vi "Crossover v2.vi"(10 "Path In 2":T1={"Distance"=0.0, "Tour"=[1, 8, 6, 10, 4, 13, 16, 2, 3, 12, 15, 5, 9, 11, 14, 7, 1]}, 11 "Path In 1":T1={"Distance"=0.0, "Tour"=[1, 14, 13, 12, 7, 6, 15, 5, 11, 9, 10, 16, 3, 2, 4, 8, 1]}) -> (2 "Path Out 2":T1, 3 "Path Out 1":T1)   [LabVIEW 2015, in "TSP Library.lvlib"]
uses:
  TSP Library.lvlib
  TypeDef/Path.ctl
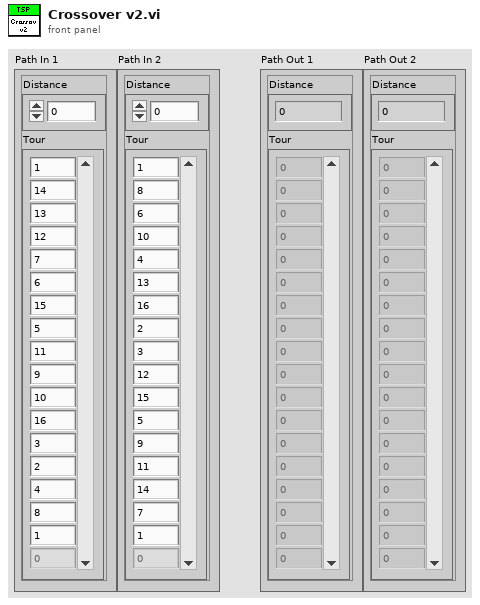
[diagram p1: front panel]
types:
  T1 = typedef "TSP Library.lvlib/Path.ctl" = cluster{"Distance":dbl, "Tour":u16[]}
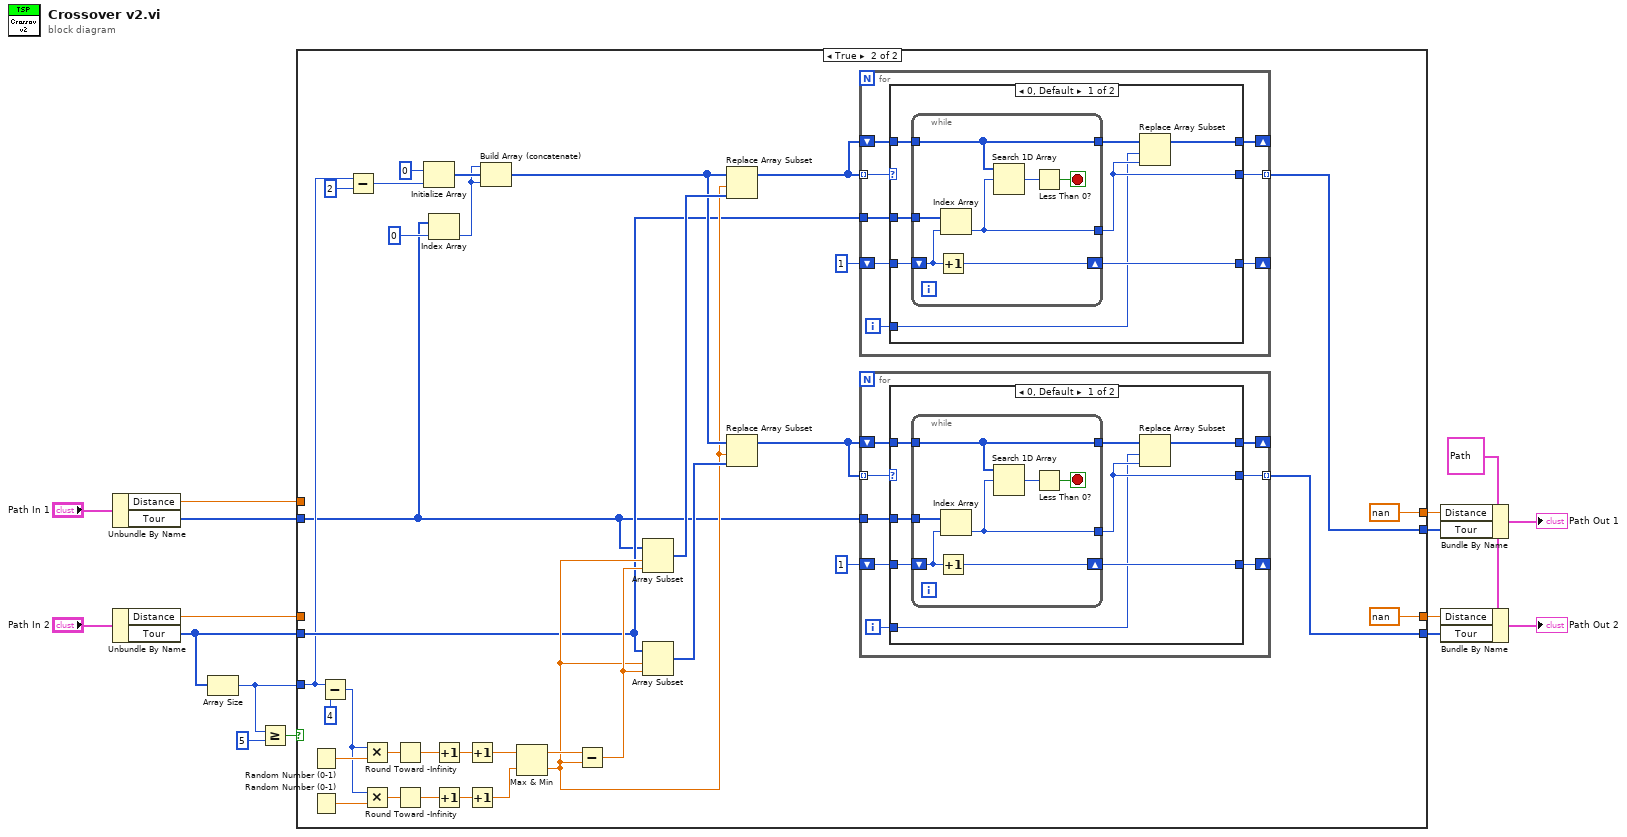
[diagram p0: block diagram]
diagram:
  w9 = T1 {"Distance"=0.0, "Tour"=[68, 82, 14, 66, 38, 76, 91, 89, 87, 84, 25, 25, 88]} ("Path In 1")
  n1 = Unbundle By Name("Path In 1") -> ("Distance"=w11:dbl, "Tour"=w12:u16[])
  n2 = Unbundle By Name("Path In 2") -> ("Distance"=w13:dbl, "Tour"=w14:u16[])
  n3 = Array Size(array=w14) -> (size(s)=w2:i32)
  n4 = Greater Or Equal?(x=w2, y=5) -> (x >= y?=w3:bool)
  n5 = case shown="True" w3 {
    tunnel: w2 -> [_ w27]
    tunnel: w14 -> [w17 w30]
    tunnel: w13 -> [w18 _]
    tunnel: w12 -> [w19 w22]
    tunnel: w11 -> [w20 _]
    tunnel: [w19 w25] -> w7
    tunnel: [w17 w21] -> w6
    tunnel: [w18 nan ("Distance")] -> w5
    tunnel: [w20 nan ("Distance")] -> w4
    frame False {
    }
    frame True {
      n6 = Random Number (0-1)() -> (number: 0 to 1=w54:dbl)
      n7 = Random Number (0-1)() -> (number: 0 to 1=w55:dbl)
      n8 = Subtract(x=w27, y=4) -> (x-y=w45:i32)
      n9 = Subtract(x=w27, y=2) -> (x-y=w28:i32)
      n10 = Multiply(x=w45, y=w54) -> (x*y=w53:dbl)
      n11 = Multiply(x=w45, y=w55) -> (x*y=w52:dbl)
      n12 = Round Toward -Infinity(1:w53) -> (0:w51:dbl)
      n13 = Round Toward -Infinity(1:w52) -> (0:w50:dbl)
      n14 = Initialize Array(u16 0 ("Numeric"), w28) -> (w37:u16[])
      n15 = Index Array(array=w22, index=0) -> (element=w36:u16)
      n16 = Increment(x=w51) -> (x+1=w43:dbl)
      n17 = Increment(x=w50) -> (x+1=w42:dbl)
      n18 = Increment(x=w43) -> (x+1=w41:dbl)
      n19 = Increment(x=w42) -> (x+1=w40:dbl)
      n20 = Build Array (concatenate)(w36, w37, w36) -> (w34:u16[])
      n21 = Max & Min(x=w41, y=w40) -> (max(x,y)=w49:dbl, min(x,y)=w32:dbl)
      n22 = Subtract(x=w49, y=w32) -> (x-y=w48:dbl)
      n23 = Array Subset(array=w22, index=w32, length=w48) -> (w35:u16[])
      n24 = Array Subset(array=w30, index=w32, length=w48) -> (w33:u16[])
      n25 = Replace Array Subset(array=w34, new element=w35, index=w32) -> (w29:u16[])
      n26 = Replace Array Subset(array=w34, new element=w33, index=w32) -> (w23:u16[])
      n27 = for {
        tunnel: w29 -> [w89] mode=indexing
        tunnel: [w88] -> w25 mode=indexing
        shift-right: [w84] -> _
        shift-left: 1 -> [w85]
        tunnel: w30 -> [w87]
        shift-right: [w83] -> _
        shift-left: w29 -> [w86]
        i -> [w82]
        n28 = case shown="0, Default" w89 {
          selector: w89 -> [_ w107]
          tunnel: [w92 w107] -> w88
          tunnel: w87 -> [w96 _]
          tunnel: w86 -> [w95 w105]
          tunnel: w85 -> [w97 w106]
          tunnel: [w94 w106] -> w84
          tunnel: [w91 w105] -> w83
          tunnel: w82 -> [w90 _]
          frame 0, Default {
            n29 = while {
              tunnel: w96 -> [w104]
              tunnel: w95 -> [w99]
              shift-right: [w102] -> w94
              shift-left: w97 -> [w103]
              tunnel: [w99] -> w93
              tunnel: [w98] -> w92
              stop <- w100 stop-if-true
              n30 = Increment(x=w103) -> (x+1=w102:i32)
              n31 = Index Array(array=w104, index=w103) -> (element=w98:u16)
              n32 = Search 1D Array(1D array=w99, element=w98) -> (index of element=w101:i32)  [unwired: 1 in]
              n33 = Less Than 0?(x=w101) -> (x < 0?=w100:bool)
            }
            n34 = Replace Array Subset(array=w93, new element=w92, index=w90) -> (w91:u16[])
          }
          frame 1.. {
          }
        }
      }
      n35 = for {
        tunnel: w23 -> [w63] mode=indexing
        tunnel: [w62] -> w21 mode=indexing
        shift-right: [w58] -> _
        shift-left: 1 -> [w59]
        tunnel: w22 -> [w61]
        shift-right: [w57] -> _
        shift-left: w23 -> [w60]
        i -> [w56]
        n36 = case shown="0, Default" w63 {
          selector: w63 -> [_ w81]
          tunnel: [w66 w81] -> w62
          tunnel: w61 -> [w70 _]
          tunnel: w60 -> [w69 w79]
          tunnel: w59 -> [w71 w80]
          tunnel: [w68 w80] -> w58
          tunnel: [w65 w79] -> w57
          tunnel: w56 -> [w64 _]
          frame 0, Default {
            n37 = while {
              tunnel: w70 -> [w78]
              tunnel: w69 -> [w73]
              shift-right: [w76] -> w68
              shift-left: w71 -> [w77]
              tunnel: [w73] -> w67
              tunnel: [w72] -> w66
              stop <- w74 stop-if-true
              n38 = Increment(x=w77) -> (x+1=w76:i32)
              n39 = Index Array(array=w78, index=w77) -> (element=w72:u16)
              n40 = Search 1D Array(1D array=w73, element=w72) -> (index of element=w75:i32)  [unwired: 1 in]
              n41 = Less Than 0?(x=w75) -> (x < 0?=w74:bool)
            }
            n42 = Replace Array Subset(array=w67, new element=w66, index=w64) -> (w65:u16[])
          }
          frame 1.. {
          }
        }
      }
    }
  }
  n43 = Bundle By Name(cluster=w9, "Distance"=w4, "Tour"=w7) -> (→"Path Out 1":T1)
  n44 = Bundle By Name(cluster=w9, "Distance"=w5, "Tour"=w6) -> (→"Path Out 2":T1)
